vi "Initialize Settings from File.vi"(8 "error in (no error)":errorcluster, 11 "SDF Path":path) -> (0 "error out":errorcluster, 1 "Visible?":bool, 2 "Channels":string[](array[string]), 3 "Rate":i32)   [LabVIEW 2015]
uses:
  <vilib>/Utility/config.llb/Read Key (Boolean).vi
  <vilib>/Utility/config.llb/Read Key (I32).vi
  <vilib>/Utility/config.llb/Write Key (Boolean).vi
  <vilib>/Utility/config.llb/Write Key (I32).vi
  <vilib>/Utility/config.llb/NI_LVConfig.lvlib
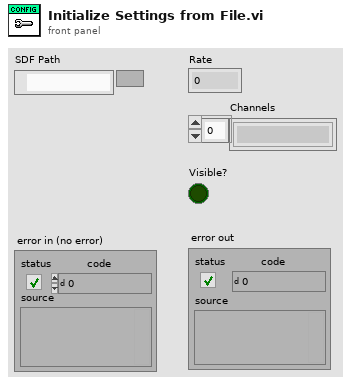
[diagram p1: front panel]
types:
  T1 = typedef "NI_LVConfig.lvlib/Config Data RefNum.ctl" = refnum<k1>
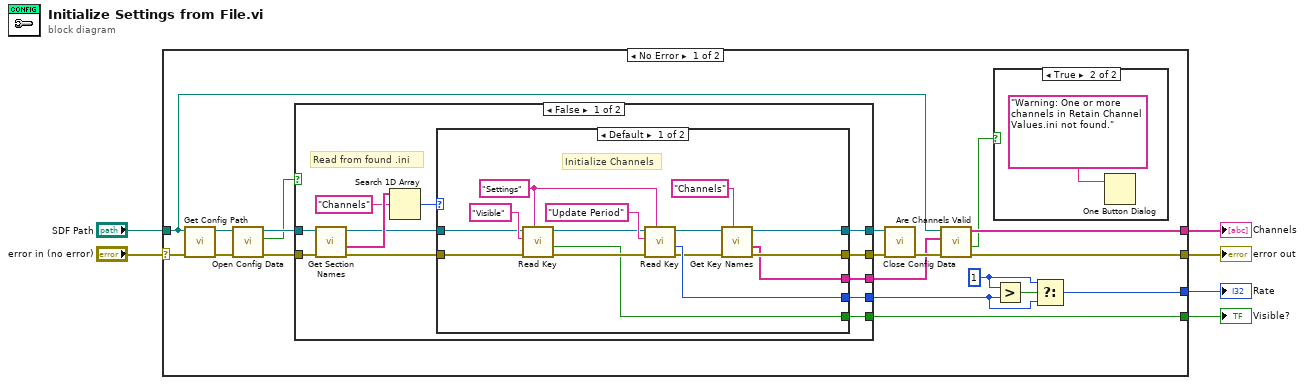
[diagram p0: block diagram]
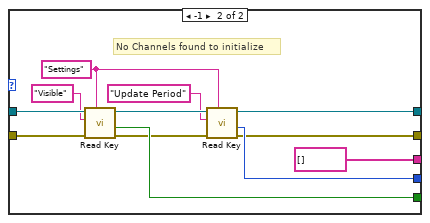
[diagram p3: hidden frame]
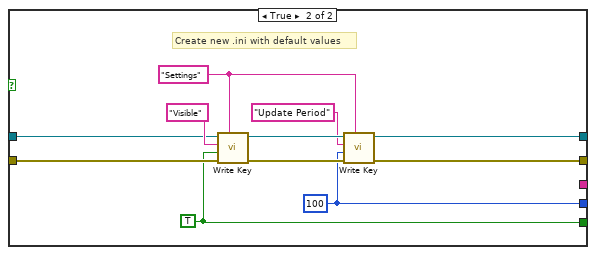
[diagram p4: hidden frame]
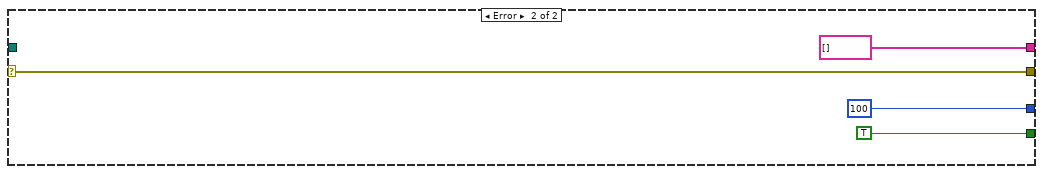
[diagram p5: hidden frame]
diagram:
  n1 = case shown="No Error" "error in (no error)" {
    selector: "error in (no error)" -> [w18 w80]
    tunnel: [w15 w80] -> w6
    tunnel: [w13 string[] [] ("Channels")] -> w5
    tunnel: [w23 TRUE ("value")] -> w4
    tunnel: [w7 100 ("value")] -> w3
    tunnel: "SDF Path" -> [w12 _]
    frame No Error {
      w9 = 1 ("x")
      n2 = call "Get Config Path.vi"("error in (no error)"=w18, "Sys Def Path"=w12) -> ("error out"=w17:errorcluster, "Config Path"=w19:path)  [unwired: 8 in]
      n3 = call <vilib>:"Open Config Data.vi"("error in (no error)"=w17, "configuration file path"=w19) -> ("error out"=w24:errorcluster, "file created?"=w20:bool, "refnum"=w25:T1)  [unwired: 7 in]
      n4 = case shown="False" w20 {
        tunnel: w25 -> [w38 w69]
        tunnel: w24 -> [w37 w68]
        tunnel: [w31 _] -> w14
        tunnel: [w30 w66] -> w23
        tunnel: [w29 w67] -> w8
        tunnel: [w28 w70] -> w22
        tunnel: [w27 w71] -> w21
        frame False {
          # "Read from found .ini"
          n5 = call <vilib>:"Get Section Names.vi"("error in (no error)"=w37, "refnum"=w38) -> ("error out"=w32:errorcluster, "section names"=w36:string[], "refnum out"=w33:T1)  [unwired: 7 in]
          n6 = Search 1D Array(1D array=w36, element="Channels") -> (index of element=w34:i32)  [unwired: 1 in]
          n7 = case shown="Default" w34 {
            tunnel: w33 -> [w47 w62]
            tunnel: w32 -> [w48 w64]
            tunnel: [w39 string[] [] ("Channels")] -> w31
            tunnel: [w46 w59] -> w30
            tunnel: [w45 w56] -> w29
            tunnel: [w41 w55] -> w28
            tunnel: [w40 w54] -> w27
            frame Default {
              w49 = "Settings" ("element")
              # "Initialize Channels"
              n8 = call-poly <vilib>:"Read Key.vi"("section"=w49, "error in (no error)"=w48, "key"="Visible" ("element"), "refnum"=w47) -> ("error out"=w52:errorcluster, "value"=w46:bool, "refnum out"=w50:T1)  [unwired: 4 in, 1 out]
              n9 = call-poly <vilib>:"Read Key.vi"("section"=w49, "error in (no error)"=w52, "key"="Update Period" ("element"), "refnum"=w50) -> ("error out"=w42:errorcluster, "value"=w45:i32, "refnum out"=w43:T1)  [unwired: 4 in, 1 out]
              n10 = call <vilib>:"Get Key Names.vi"("section"="Channels" ("element"), "error in (no error)"=w42, "refnum"=w43) -> ("error out"=w41:errorcluster, "key names"=w39:string[], "refnum out"=w40:T1)  [unwired: 5 in, 1 out]
            }
            frame -1 {
              w63 = "Settings" ("element")
              # "No Channels found to initialize"
              n11 = call-poly <vilib>:"Read Key.vi"("section"=w63, "error in (no error)"=w64, "key"="Visible" ("element"), "refnum"=w62) -> ("error out"=w58:errorcluster, "value"=w59:bool, "refnum out"=w61:T1)  [unwired: 4 in, 1 out]
              n12 = call-poly <vilib>:"Read Key.vi"("section"=w63, "error in (no error)"=w58, "key"="Update Period" ("element"), "refnum"=w61) -> ("error out"=w55:errorcluster, "value"=w56:i32, "refnum out"=w54:T1)  [unwired: 4 in, 1 out]
            }
          }
        }
        frame True {
          w67 = 100
          w66 = TRUE ("value")
          w73 = "Settings" ("section")
          # "Create new .ini with default values"
          n13 = call-poly <vilib>:"Write Key.vi"("section"=w73, "error in (no error)"=w68, "value"=w66, "key"="Visible", "refnum"=w69) -> ("error out"=w76:errorcluster, "refnum out"=w74:T1)  [unwired: 4 in, 1 out]
          n14 = call-poly <vilib>:"Write Key.vi"("section"=w73, "error in (no error)"=w76, "value"=w67, "key"="Update Period", "refnum"=w74) -> ("error out"=w70:errorcluster, "refnum out"=w71:T1)  [unwired: 4 in, 1 out]
        }
      }
      n15 = call <vilib>:"Close Config Data.vi"("error in (no error)"=w22, "refnum"=w21) -> ("error out"=w16:errorcluster)  [unwired: 8 in, 1 out]
      n16 = call "Are Channels Valid.vi"("error in (no error)"=w16, "Channels In"=w14, "SDF Path"=w12) -> ("error out"=w15:errorcluster, "Invalid Channels Found?"=w11:bool, "Valid Channels Out"=w13:string[])  [unwired: 5 in, 1 out]
      n17 = case shown="True" w11 {
        frame False {
        }
        frame True {
          n18 = One Button Dialog(message="Warning: One or more channels in Retain Channel Values.ini not found.") -> ()  [unwired: 1 in, 1 out]
        }
      }
      n19 = Greater?(x=w9, y=w8) -> (0:w10:bool)
      n20 = Select(t=w9, s=w10, f=w8) -> (s? t:f=w7:i32)
    }
    frame Error {
    }
  }
  "error out" <- w6
  "Channels" <- w5
  "Rate" <- w3
  "Visible?" <- w4
